vi "PotMotorMain.vi"() -> ()   [LabVIEW 2014]
uses:
  <vilib>/myRIO/Instrument Drivers/Onboard IO/PWM/typedefs/PWM Reference.ctl
  <vilib>/myRIO/Common/Instrument Driver Framework/Utilities/typedefs/myRIO Generic Hardware Reference.ctl
  <vilib>/myRIO/Common/Instrument Driver Framework/Utilities/typedefs/Hardware Version Enum.ctl
  <vilib>/myRIO/Common/Instrument Driver Framework/Utilities/typedefs/myRIO v1.0 Reference.ctl
  <vilib>/myRIO/Common/Instrument Driver Framework/Utilities/typedefs/Generic FPGA Reference.ctl
  <vilib>/myRIO/Common/Instrument Driver Framework/myRIO v1.0/PWM/typedefs/PWM Channels Enum.ctl
  <vilib>/myRIO/Instrument Drivers/Onboard IO/PWM/typedefs/PWM Configuration.ctl
  <vilib>/userdefined/High Color/nirio_resource_hc.ctl
  <vilib>/myRIO/Instrument Drivers/Onboard IO/AI/typedefs/AI Reference.ctl
  <vilib>/myRIO/Common/Instrument Driver Framework/myRIO v1.0/AI/typedefs/AI Channels List.ctl
  <vilib>/myRIO/Common/Instrument Driver Framework/myRIO v1.0/AI/typedefs/AI Channels Enum.ctl
  <vilib>/myRIO/Common/Instrument Driver Framework/Utilities/typedefs/Analog Scaling Constants List.ctl
  <vilib>/myRIO/Common/Instrument Driver Framework/Utilities/typedefs/Analog Scaling Constants.ctl
  <vilib>/myRIO/Common/Instrument Driver Framework/myRIO v1.0/PWM/vis/myRIO v1.1 Open PWM.vi
  <vilib>/myRIO/Common/Instrument Driver Framework/myRIO v1.0/AI/vis/myRIO v1.1 Open AI.vi
  <vilib>/myRIO/Common/Instrument Driver Framework/Utilities/vis/Validate Channels.vi
  <vilib>/myRIO/Common/Instrument Driver Framework/myRIO v1.0/PWM/vis/myRIO v1.0 Reserve PWM.vi
  <vilib>/myRIO/Instrument Drivers/Onboard IO/PWM/vis/Set Duty Cycle and Frequency.vi
  <vilib>/myRIO/Common/Instrument Driver Framework/myRIO v1.0/AI/vis/myRIO v1.0 Reserve AI.vi
  <vilib>/myRIO/Common/Instrument Driver Framework/myRIO v1.0/DIO/vis/myRIO v1.1 Open DIO.vi
  <vilib>/myRIO/Common/Instrument Driver Framework/myRIO v1.0/PWM/vis/myRIO v1.0 Close PWM.vi
  <vilib>/myRIO/Common/Instrument Driver Framework/myRIO v1.0/AI/vis/myRIO v1.0 Close AI.vi
  <vilib>/myRIO/Common/Instrument Driver Framework/myRIO v1.0/DIO/vis/myRIO v1.0 Close DIO.vi
  <vilib>/myRIO/Common/Instrument Driver Framework/myRIO v1.0/PWM/vis/myRIO v1.0 Build MUX Configuration PWM.vi
  <vilib>/myRIO/Common/Instrument Driver Framework/myRIO v1.0/Resource Manager/vis/myRIO v1.0 Reserve Channel List.vi
  <vilib>/myRIO/Common/Instrument Driver Framework/myRIO v1.0/AI/vis/myRIO v1.0 Build MUX Configuration AI.vi
  <vilib>/myRIO/Common/Instrument Driver Framework/myRIO v1.0/DIO/vis/myRIO v1.0 Reserve DIO.vi
  <vilib>/myRIO/Common/Instrument Driver Framework/myRIO v1.0/PWM/vis/myRIO v1.0 Unreserve PWM.vi
  <vilib>/myRIO/Common/Instrument Driver Framework/myRIO v1.0/AI/vis/myRIO v1.0 Unreserve AI.vi
  <vilib>/myRIO/Common/Instrument Driver Framework/myRIO v1.0/DIO/vis/myRIO v1.0 Unreserve DIO.vi
  <vilib>/myRIO/Common/Instrument Driver Framework/myRIO v1.0/Resource Manager/vis/myRIO v1.0 Create Configuration List.vi
  <vilib>/myRIO/Common/Instrument Driver Framework/myRIO v1.0/Resource Manager/vis/myRIO v1.0 Reserve Channel.vi
  <vilib>/myRIO/Common/Instrument Driver Framework/myRIO v1.0/Resource Manager/vis/myRIO v1.0 Unreserve Channel.vi
  <vilib>/myRIO/Common/Instrument Driver Framework/myRIO v1.0/DIO/vis/myRIO v1.0 Build MUX Configuration DIO.vi
  <vilib>/myRIO/Common/Instrument Driver Framework/myRIO v1.0/Resource Manager/vis/myRIO v1.0 Unreserve Channel List.vi
  <vilib>/myRIO/Common/Instrument Driver Framework/myRIO v1.0/Resource Manager/vis/myRIO v1.0 Build Mutex Name.vi
  <vilib>/Utility/VariantDataType/GetNumericInfo.vi
  <vilib>/Utility/error.llb/Error Cluster From Error Code.vi
  <vilib>/myRIO/Common/Instrument Driver Framework/myRIO v1.0/myRIO v1.1 Open.vi
  <vilib>/myRIO/Common/Instrument Driver Framework/Utilities/vis/IO Manager.vi
  <vilib>/myRIO/Common/Instrument Driver Framework/Utilities/vis/Configuration Manager.vi
  <vilib>/myRIO/Common/Instrument Driver Framework/myRIO v1.0/Resource Manager/vis/myRIO v1.0 Configure IO.vi
  <vilib>/myRIO/Common/Instrument Driver Framework/myRIO v1.0/myRIO v1.0 Close.vi
  <vilib>/myRIO/Common/Instrument Driver Framework/myRIO v1.0/AI/vis/myRIO v1.0 Get Scaling Constants AI.vi
  <vilib>/myRIO/Common/Instrument Driver Framework/myRIO v1.0/PWM/vis/myRIO v1.0 Write PWM.vi
  <vilib>/myRIO/Common/Instrument Driver Framework/myRIO v1.0/PWM/vis/myRIO v1.0 Shutdown PWM.vi
  <vilib>/myRIO/Common/Instrument Driver Framework/myRIO v1.0/AI/vis/myRIO v1.0 Read AI.vi
  <vilib>/myRIO/Common/Instrument Driver Framework/myRIO v1.0/DIO/vis/myRIO v1.0 Write DIO.vi
  <vilib>/myRIO/Common/Instrument Driver Framework/myRIO v1.0/DIO/vis/myRIO v1.0 Shutdown DIO.vi
  <vilib>/myRIO/Instrument Drivers/Onboard IO/AI/vis/myRIO AI Open.xnode
  <vilib>/myRIO/Instrument Drivers/Onboard IO/PWM/vis/myRIO PWM Open.xnode
  <vilib>/myRIO/Instrument Drivers/Onboard IO/DIO/DIO.lvlib
  <vilib>/myRIO/Instrument Drivers/Onboard IO/AI/AI.lvlib
  <vilib>/myRIO/Instrument Drivers/Onboard IO/PWM/PWM.lvlib
  <vilib>/gmath/NI_Gmath.lvlib
panel:
  in  "Pot. Degrees":dbl[](array[numeric])
  in  "Propmotor PWM Channel":tag="C/PWM1"
  in  "Servo PWM Channel":tag="C/PWM0"
  out "error out":errorcluster
  out "Volts":dbl(knob) scale=0.0..10.0
  out "Active":bool
  in  "Stop":bool
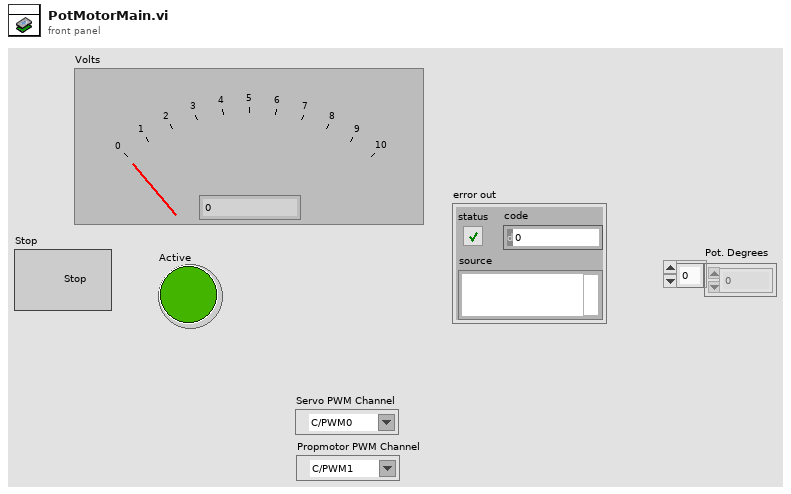
[diagram p1: front panel]
types:
  T1 = typedef "nirio_resource_hc.ctl" = tag
  T2 = typedef "Hardware Version Enum.ctl" = enum16{"Unknown", "myRIO-1900", "myRIO-1950"}
  T3 = typedef "PWM.lvlib/PWM Reference.ctl" = cluster{"myRIO Reference":T4, "PWM Channels Enum":T7, "PWM Configuration":T8}
  T4 = typedef "myRIO Generic Hardware Reference.ctl" = cluster{"myRIO Model":T2, "myRIO Hardware Reference":T5}
  T5 = typedef "myRIO v1.0 Reference.ctl" = cluster{"Generic FPGA Reference":T6, "Allow multiple opens":bool}
  T6 = typedef "Generic FPGA Reference.ctl" = refnum<k20>
  T7 = typedef "PWM Channels Enum.ctl" = enum16{"Not Connected", "C/PWM0", "C/PWM1", "A/PWM0", "A/PWM1", "A/PWM2", "B/PWM0", "B/PWM1", "B/PWM2"}
  T8 = typedef "PWM.lvlib/PWM Configuration.ctl" = cluster{"Frequency":dbl, "Duty Cycle":dbl}
  T9 = typedef "DIO.lvlib/DIO Reference.ctl" = cluster{"myRIO Reference":T4, "DIO Channels List":T10}
  T10 = typedef "DIO Channels List.ctl" = T11[]
  T11 = typedef "DIO Channels Enum.ctl" = enum16{"Not Connected", "C/DIO0", "C/DIO1", "C/DIO2", "C/DIO3", "C/DIO4", "C/DIO5", "C/DIO6", "C/DIO7", "A/DIO0", "A/DIO1", "A/DIO2", "A/DIO3", "A/DIO4", "A/DIO5", "A/DIO6", "A/DIO7", "A/DIO8", "A/DIO9", "A/DIO10", "A/DIO11", "A/DIO12", "A/DIO13", "A/DIO14", "A/DIO15", "B/DIO0", "B/DIO1", "B/DIO2", "B/DIO3", "B/DIO4", "B/DIO5", "B/DIO6", "B/DIO7", "B/DIO8", "B/DIO9", "B/DIO10", "B/DIO11", "B/DIO12", "B/DIO13", "B/DIO14", "B/DIO15", "LED0", "LED1", "LED2", "LED3", "Button0"}
  T12 = typedef "AI.lvlib/AI Reference.ctl" = cluster{"myRIO Reference":T4, "AI Channels List":T13, "AI Scaling Constants List":T15}
  T13 = typedef "AI Channels List.ctl" = T14[]
  T14 = typedef "AI Channels Enum.ctl" = enum16{"Not Connected", "AudioIn/Left", "AudioIn/Right", "C/AI0", "C/AI1", "A/AI0", "A/AI1", "A/AI2", "A/AI3", "B/AI0", "B/AI1", "B/AI2", "B/AI3"}
  T15 = typedef "Analog Scaling Constants List.ctl" = T16[]
  T16 = typedef "Analog Scaling Constants.ctl" = cluster{"LSB Weight (Volts)":dbl, "Offset (Volts)":dbl, "Signed?":bool}
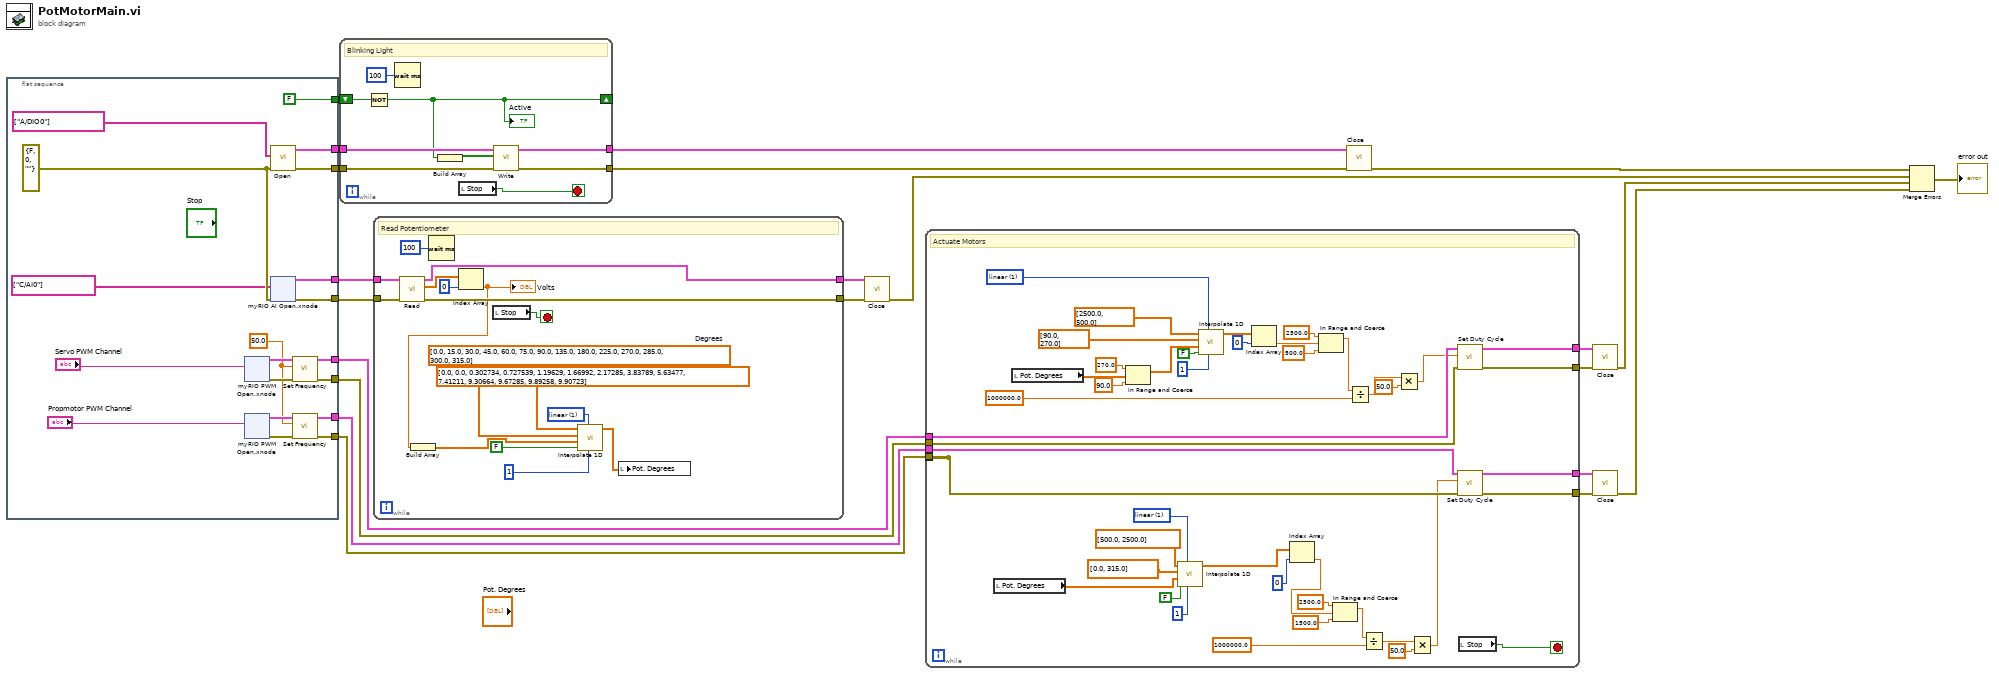
[diagram p0: block diagram]
diagram:
  n1 = flat-sequence {
    tunnel: [w39] -> w21
    tunnel: [w38] -> w20
    tunnel: [FALSE] -> w22
    tunnel: [w36] -> w18
    tunnel: [w35] -> w19
    tunnel: [w26] -> w10
    tunnel: [w25] -> w9
    tunnel: [w24] -> w8
    tunnel: [w23] -> w7
    frame #0 {
      w27 = 50.0 ("Frequency [Hz]")
      w41 = errorcluster {"status"=FALSE, "code"=0, "source"=""} ("error out")
      n2 = xnode "myRIO PWM Open.xnode"("Channel Name"="Servo PWM Channel") -> ("error out"=w32:errorcluster, "PWM Ref Out"=w33:T3)  [unwired: 2 in]
      n3 = xnode "myRIO PWM Open.xnode"("Channel Name"="Propmotor PWM Channel") -> ("error out"=w29:errorcluster, "PWM Ref Out"=w30:T3)  [unwired: 2 in]
      n4 = call <vilib>:"Open.vi"("error in (no error)"=w41, "Channel Names"=tag[] ["A/DIO0"]) -> ("error out"=w38:errorcluster, "DIO Ref Out"=w39:T9)  [unwired: 8 in]
      n5 = xnode "myRIO AI Open.xnode"("error in (no error)"=w41, "Channel Names"=tag[] ["C/AI0"]) -> ("error out"=w36:errorcluster, "AI Ref Out"=w35:T12)  [unwired: 1 in]
      n6 = call <vilib>:"Set Frequency.vi"("error in (no error)"=w32, "Frequency [Hz]"=w27, "PWM Ref In"=w33) -> ("error out"=w25:errorcluster, "PWM Ref Out"=w26:T3)  [unwired: 6 in]
      n7 = call <vilib>:"Set Frequency.vi"("error in (no error)"=w29, "Frequency [Hz]"=w27, "PWM Ref In"=w30) -> ("error out"=w23:errorcluster, "PWM Ref Out"=w24:T3)  [unwired: 6 in]
    }
  }
  n8 = while {
    shift-right: [w92] -> _
    shift-left: w22 -> [w98]
    tunnel: w21 -> [w97]
    tunnel: w20 -> [w96]
    tunnel: [w95] -> w16
    tunnel: [w94] -> w17
    stop <- w99 stop-if-true
    # "Blinking Light"
    n9 = Not(x=w98) -> (.not. x?=w92:bool)
    "Active" <- w92
    n10 = Wait (ms)(milliseconds to wait=u32 100) -> ()  [unwired: 1 out]
    n11 = Build Array(w92) -> (w93:bool[])
    n12 = local read "Stop"() -> (w99:bool)
    n13 = call <vilib>:"Write.vi"("error in (no error)"=w96, "Values"=w93, "DIO Ref In"=w97) -> ("error out"=w95:errorcluster, "DIO Ref Out"=w94:T9)  [unwired: 6 in]
  }
  n14 = while {
    tunnel: w19 -> [w114]
    tunnel: w18 -> [w113]
    tunnel: [w110] -> w15
    tunnel: [w109] -> w11
    stop <- w115 stop-if-true
    w101 = dbl[] [0.0, 15.0, 30.0, 45.0, 60.0, 75.0, 90.0, 135.0, 180.0, 225.0, 270.0, 285.0, 300.0, 315.0]  # Degrees
    w104 = 1 items=["nearest", "linear", "spline", "cubic Hermite", "Lagrange"] ("method")
    # "Read Potentiometer"
    n15 = call <vilib>:"Read.vi"("error in (no error)"=w113, "AI Ref In"=w114) -> ("error out"=w110:errorcluster, "Values"=w112:dbl[], "AI Ref Out"=w109:T12)  [unwired: 7 in]
    n16 = Wait (ms)(milliseconds to wait=u32 100) -> ()  [unwired: 1 out]
    n17 = Index Array(array=w112, index=0) -> (element=w107:dbl)
    "Volts" <- w107
    n18 = Build Array(w107) -> (w106:dbl[])
    n19 = local read "Stop"() -> (w115:bool)
    n20 = call <vilib>:"Interpolate 1D.vi"("ntimes"=1, "method"=w104, "X is monotonic"=FALSE, "xi"=w106, "X"=dbl[] [0.0, 0.0, 0.302734, 0.727539, 1.19629, 1.66992, 2.17285, 3.83789, 5.63477, 7.41211, 9.30664, 9.67285, 9.89258, 9.90723] ("VoltageIn"), "Y"=w101) -> ("yi"=w102:dbl[])  [unwired: 3 in, 2 out]
    n21 = local write "Pot. Degrees"(w102) -> ()
  }
  n22 = call <vilib>:"Close.vi"("error in (no error)"=w15, "AI Ref In"=w11) -> ("error out"=w13:errorcluster)  [unwired: 9 in]
  n23 = while {
    tunnel: w10 -> [w159]
    tunnel: w9 -> [w158]
    tunnel: w8 -> [w157]
    tunnel: [w156] -> _
    tunnel: w7 -> [w156]
    tunnel: [w155] -> w6
    tunnel: [w154] -> w5
    tunnel: [w153] -> w4
    tunnel: [w152] -> w3
    stop <- w160 stop-if-true
    w120 = 1 items=["nearest", "linear", "spline", "cubic Hermite", "Lagrange"] ("method")
    w144 = 1 items=["nearest", "linear", "spline", "cubic Hermite", "Lagrange"] ("method")
    # "Actuate Motors"
    n24 = local read "Pot. Degrees"() -> (w123:dbl[])
    n25 = local read "Pot. Degrees"() -> (w135:dbl[])
    n26 = In Range and Coerce(upper limit=270.0, x=w135, lower limit=90.0) -> (coerced(x)=w140:dbl[])  [unwired: 1 out]
    n27 = call <vilib>:"Interpolate 1D.vi"("ntimes"=1, "method"=w120, "X is monotonic"=FALSE, "xi"=w123, "X"=dbl[] [0.0, 315.0] ("X servo (degrees)"), "Y"=dbl[] [500.0, 2500.0] ("Y servo (PWM)")) -> ("yi"=w119:dbl[])  [unwired: 3 in, 2 out]
    n28 = call <vilib>:"Interpolate 1D.vi"("ntimes"=1, "method"=w144, "X is monotonic"=FALSE, "xi"=w140, "X"=dbl[] [90.0, 270.0] ("X servo (degrees)"), "Y"=dbl[] [2500.0, 500.0] ("Y servo (PWM)")) -> ("yi"=w139:dbl[])  [unwired: 3 in, 2 out]
    n29 = Index Array(array=w139, index=0) -> (element=w138:dbl)
    n30 = Index Array(array=w119, index=0) -> (element=w118:dbl)
    n31 = In Range and Coerce(upper limit=2500.0, x=w138, lower limit=500.0) -> (coerced(x)=w148:dbl)  [unwired: 1 out]
    n32 = In Range and Coerce(upper limit=2500.0, x=w118, lower limit=1500.0) -> (coerced(x)=w131:dbl)  [unwired: 1 out]
    n33 = Divide(x=w148, y=1000000.0) -> (x/y=w146:dbl)
    n34 = Divide(x=w131, y=1000000.0) -> (x/y=w128:dbl)
    n35 = Multiply(x=w146, y=50.0) -> (x*y=w126:dbl)
    n36 = Multiply(x=w128, y=50.0) -> (x*y=w127:dbl)
    n37 = call <vilib>:"Set Duty Cycle.vi"("error in (no error)"=w158, "Duty Cycle"=w126, "PWM Ref In"=w159) -> ("error out"=w154:errorcluster, "PWM Ref Out"=w155:T3)  [unwired: 6 in]
    n38 = call <vilib>:"Set Duty Cycle.vi"("error in (no error)"=w156, "Duty Cycle"=w127, "PWM Ref In"=w157) -> ("error out"=w153:errorcluster, "PWM Ref Out"=w152:T3)  [unwired: 6 in]
    n39 = local read "Stop"() -> (w160:bool)
  }
  n40 = call <vilib>:"Close.vi"("error in (no error)"=w16, "DIO Ref In"=w17) -> ("error out"=w14:errorcluster)  [unwired: 9 in]
  n41 = call <vilib>:"Close.vi"("error in (no error)"=w5, "PWM Ref In"=w6) -> ("error out"=w2:errorcluster)  [unwired: 9 in]
  n42 = call <vilib>:"Close.vi"("error in (no error)"=w4, "PWM Ref In"=w3) -> ("error out"=w1:errorcluster)  [unwired: 9 in]
  n43 = Merge Errors(w14, w13, w2, w1) -> (→"error out":errorcluster)
